vi "Launch Digital Reader.vi"(8 "error in (no error)":errorcluster, 11 "Root Tester in":refnum<class "Root Tester.lvclass">) -> (0 "error out":errorcluster, 3 "Root Tester out":refnum<class "Root Tester.lvclass">)   [LabVIEW 2024, in "Root Tester.lvlib" / "Root Tester.lvclass"]
uses:
  Root Tester.lvclass
  <vilib>/DAQmx/create/channels.llb/DAQmx Create Channel (DI-Digital Input).vi
  DAQmx Actor/Digital Reader/Digital Reader.lvclass
  Root Tester.lvclass/Root Tester.ctl
  C:/Program Files (x86)/National Instruments/LabVIEW 2024/vi.lib/ActorFramework/Actor/Actor.lvclass
  C:/Users/uspoaotto/OneDrive - Oregon Tool/Desktop/working copies/DAQmxActor/src/Root Tester/Root Tester/Root Tester.lvclass
  C:/Users/uspoaotto/OneDrive - Oregon Tool/Desktop/working copies/DAQmxActor/src/DAQmx Actor Interface/Analog Input Waveform Data/Analog Input Waveform Data.lvclass
  C:/Users/uspoaotto/OneDrive - Oregon Tool/Desktop/working copies/DAQmxActor/src/DAQmx Actor Interface/Digital Input Data/Digital Input Data.lvclass
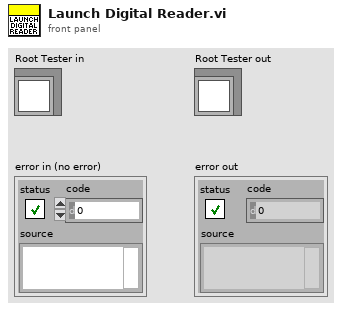
[diagram p1: front panel]
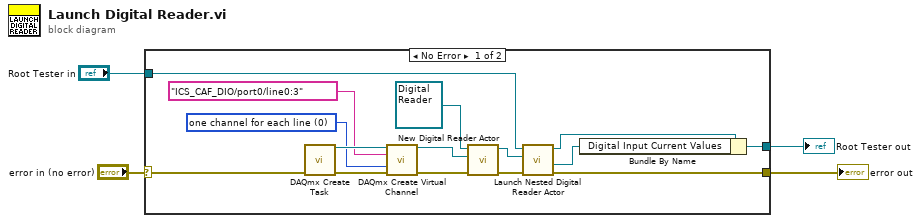
[diagram p0: block diagram]
diagram:
  n1 = case shown="No Error" "error in (no error)" {
    selector: "error in (no error)" -> [w12 w21]
    tunnel: [w9 w21] -> w3
    tunnel: [w5 w20] -> w1
    tunnel: "Root Tester in" -> [w11 w20]
    frame No Error {
      w16 = 0 items=["one channel for each line", "one channel for all lines"] ("line grouping")
      n2 = call <vilib>:"DAQmx Create Task.vi"("error in"=w12) -> ("task out"=w19:refnum<k21>, "error out"=w18:errorcluster)  [unwired: 13 in]
      n3 = call-poly <vilib>:"DAQmx Create Virtual Channel.vi"("task in"=w19, "lines"=tag "ICS_CAF_DIO/port0/line0:3", "line grouping"=w16, "error in"=w18) -> ("task out"=w15:refnum<k21>, "error out"=w13:errorcluster)  [unwired: 10 in]
      n4 = call-dynamic "New Digital Reader Actor.vi"("error in (no error)"=w13, "DAQmx Task"=w15, "Digital Reader in"=refnum<class "Digital Reader.lvclass"> refnum) -> ("error out"=w8:errorcluster, "Digital Reader out"=w10:refnum<class "Digital Reader.lvclass">)  [unwired: 7 in]
      n5 = call "Launch Nested Digital Reader Actor.vi"("error in (no error)"=w8, "Nested Digital Reader Actor"=w10, "Caller Actor in"=w11) -> ("error out"=w9:errorcluster, "Digital Input Current Values"=w6:refnum<queue>, "Caller Actor out"=w7:refnum<class "Root Tester.lvclass">)  [unwired: 5 in, 1 out]
      n6 = Bundle By Name(cluster=w7, "Digital Input Current Values"=w6) -> (w5:refnum<class "Root Tester.lvclass">)
    }
    frame Error {
    }
  }
  "error out" <- w3
  "Root Tester out" <- w1
